vi "Close Error Handles.vi"(8 "error in":errorcluster, 11 "Async in":refnum<class "VS Inline Async API.lvclass">) -> (0 "error out":errorcluster, 3 "Async out":refnum<class "VS Inline Async API.lvclass">)   [LabVIEW 2015, in "VS Inline Async API.lvlib" / "VS Inline Async API.lvclass"]
uses:
  VS Inline Async API.lvclass
  VS Inline Async API.lvclass/VS Inline Async API.ctl
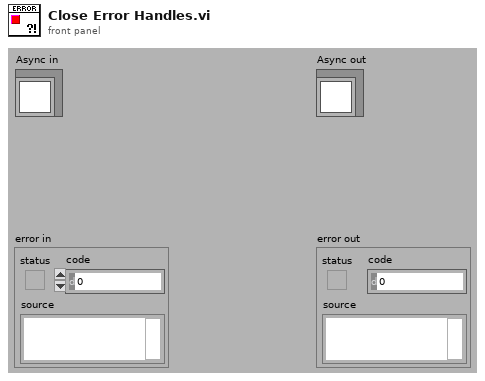
[diagram p1: front panel]
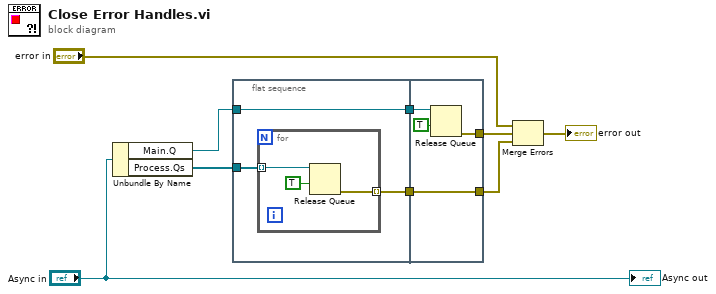
[diagram p0: block diagram]
diagram:
  n1 = Unbundle By Name("Async in") -> ("Main.Q"=w7:refnum<queue>, "Process.Qs"=w9:refnum<queue>[])
  n2 = flat-sequence {
    tunnel: w9 -> [w12]
    tunnel: [w11] -> w8
    tunnel: w7 -> [w11]
    tunnel: [w10] -> w4
    tunnel: w8 -> [w19]
    tunnel: [w18] -> w6
    tunnel: [w17] -> w5
    tunnel: w4 -> [w17]
    frame #0 {
      n3 = for {
        tunnel: w12 -> [w15] mode=indexing
        tunnel: [w14] -> w10 mode=indexing
        n4 = Release Queue(queue=w15, force destroy? (F)=TRUE) -> (error out=w14:errorcluster)  [unwired: 1 in, 2 out]
      }
    }
    frame #1 {
      n5 = Release Queue(queue=w19, force destroy? (F)=TRUE) -> (error out=w18:errorcluster)  [unwired: 1 in, 2 out]
    }
  }
  n6 = Merge Errors("error in", w6, w5) -> (→"error out":errorcluster)
  "Async out" <- "Async in"
